vi "Export.vi"(8 "error in (no error)":errorcluster, 11 "Project Path":path) -> (0 "error out":errorcluster)   [LabVIEW 2015, in "Project.lvclass"]
uses:
  Project.lvclass
  Elemental IO Properties.ctl
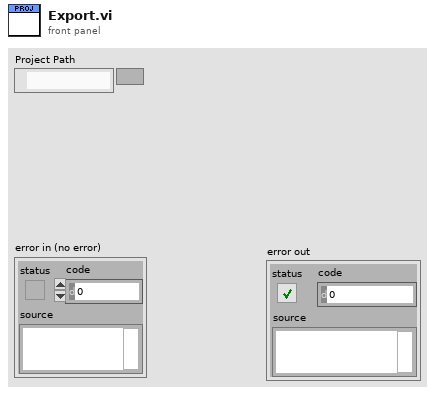
[diagram p1: front panel]
types:
  T1 = enum16{"open", "replace", "create", "open or create", "replace or create", "replace or create with confirmation"}
  T2 = typedef "Project.lvclass/Elemental IO Properties.ctl" = cluster{"FPGA":string, "Mod":string, "IO Resource":string, "IO Name":string}
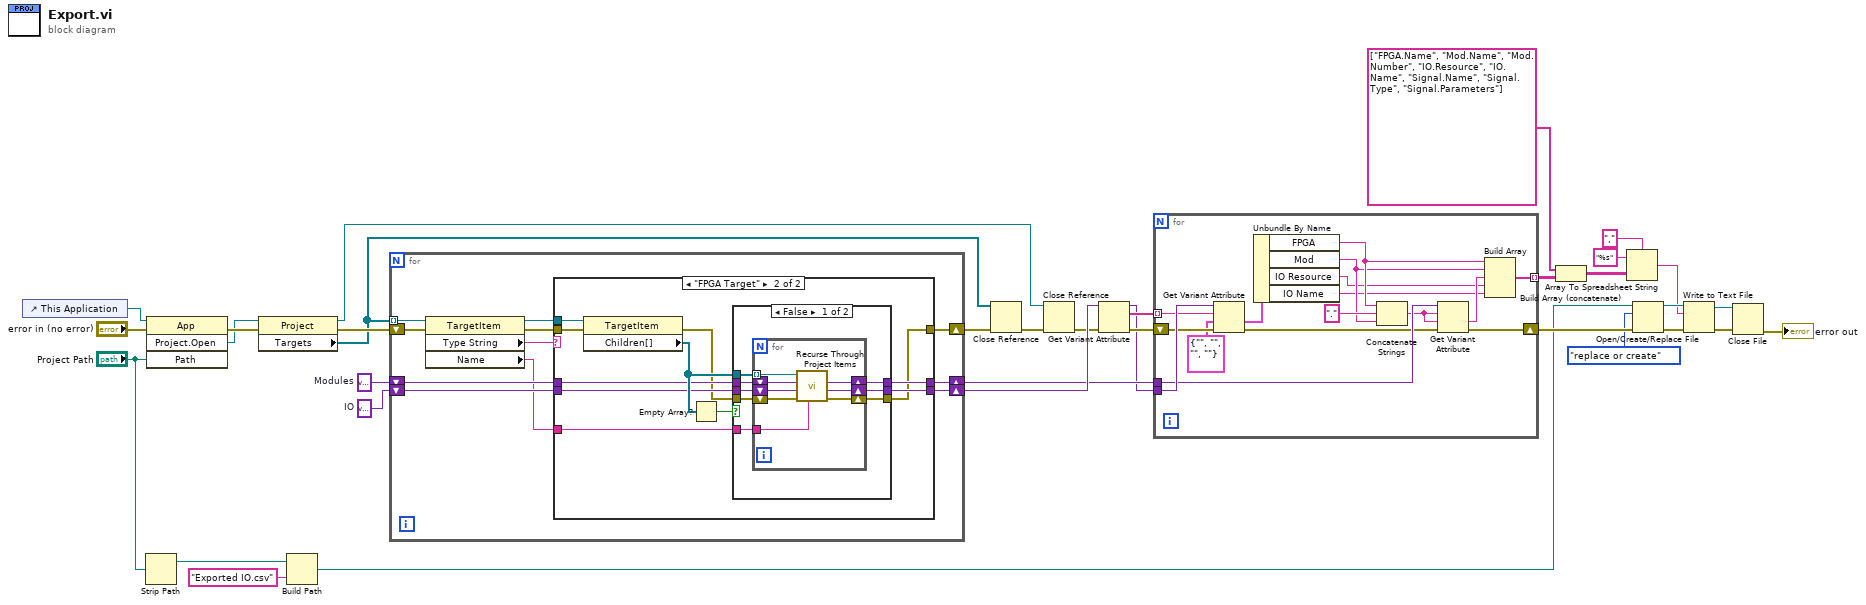
[diagram p0: block diagram]
diagram:
  w25 = variant  # IO
  w26 = variant  # Modules
  n1 = control-ref of="This Application"() -> (w34:refnum<vi>)
  n2 = Strip Path(path="Project Path") -> (stripped path=w6:path)  [unwired: 1 out]
  n3 = invoke class="App" method="Project.Open"(reference=w34, error in="error in (no error)", "Path"="Project Path") -> (error out=w33:errorcluster, "Project:Open"=w32:refnum<vi>)  [unwired: 1 in, 2 out]
  n4 = property class="Project"(reference=w32, error in=w33) -> (reference out=w28:refnum<vi>, error out=w31:errorcluster, "Targets"=w29:refnum<vi>[])
  n5 = Build Path(base path=w6, name or relative path="Exported IO.csv") -> (appended path=w3:path)
  n6 = for {
    tunnel: w29 -> [w45] mode=indexing
    shift-right: [w42] -> w30
    shift-left: w31 -> [w44]
    shift-right: [w39] -> w22
    shift-left: w26 -> [w40]
    shift-right: [w37] -> w23
    shift-left: w25 -> [w38]
    n7 = property class="TargetItem"(reference=w45, error in=w44) -> (reference out=w41:refnum<vi>, error out=w43:errorcluster, "Type String"=w36:string, "Name"=w35:string)
    n8 = case shown="\"FPGA Target\"" w36 {
      tunnel: w43 -> [w48 w59]
      tunnel: [w48 w49] -> w42
      tunnel: w41 -> [_ w58]
      tunnel: w40 -> [w47 w55]
      tunnel: w35 -> [_ w54]
      tunnel: [w47 w53] -> w39
      tunnel: w38 -> [w46 w52]
      tunnel: [w46 w51] -> w37
      frame "False", Default {
      }
      frame "FPGA Target" {
        n9 = property class="TargetItem"(reference=w58, error in=w59) -> (error out=w50:errorcluster, "Children[]"=w57:refnum<vi>[])  [unwired: 1 out]
        n10 = Empty Array?(array=w57) -> (empty?=w56:bool)
        n11 = case shown="False" w56 {
          tunnel: w57 -> [w67 _]
          tunnel: w50 -> [w66 w76]
          tunnel: w55 -> [w65 w78]
          tunnel: w54 -> [w64 _]
          tunnel: [w63 w78] -> w53
          tunnel: w52 -> [w62 w77]
          tunnel: [w61 w77] -> w51
          tunnel: [w60 w76] -> w49
          frame False {
            n12 = for {
              tunnel: w67 -> [w75] mode=indexing
              shift-right: [w73] -> w60
              shift-left: w66 -> [w74]
              shift-right: [w72] -> w63
              shift-left: w65 -> [w69]
              tunnel: w64 -> [w68]
              shift-right: [w71] -> w61
              shift-left: w62 -> [w70]
              n13 = call "Recurse Through Project Items.vi"("FPGA"=w68, "error in (no error)"=w74, "IO in"=w70, "Modules in"=w69, "ProjectItem in"=w75) -> ("error out"=w73:errorcluster, "IO out"=w71:variant, "Modules out"=w72:variant)  [unwired: 4 in]
            }
          }
          frame True {
          }
        }
      }
    }
  }
  n14 = Close Reference(reference=w29, error in (no error)=w30) -> (error out=w27:errorcluster)
  n15 = Close Reference(reference=w28, error in (no error)=w27) -> (error out=w20:errorcluster)
  n16 = Get Variant Attribute(Variant=w23, error in=w20) -> (duplicate Variant=w18:variant, names=w24:string[], error out=w21:errorcluster)  [unwired: 2 in, 1 out]
  n17 = for {
    tunnel: w24 -> [w81] mode=indexing
    tunnel: w18 -> [w94]
    tunnel: w22 -> [w93]
    tunnel: [w84] -> w1 mode=indexing
    shift-right: [w83] -> w12
    shift-left: w21 -> [w89]
    n18 = Get Variant Attribute(Variant=w94, name=w81, default value (empty Variant)=T2 {"FPGA"="", "Mod"="", "IO Resource"="", "IO Name"=""}, error in=w89) -> (value=w92:T2, error out=w90:errorcluster)  [unwired: 2 out]
    n19 = Unbundle By Name(w92) -> ("FPGA"=w88:string, "Mod"=w87:string, "IO Resource"=w85:string, "IO Name"=w80:string)
    n20 = Concatenate Strings(w88, "." ("string"), w87) -> (w82:string)
    n21 = Get Variant Attribute(Variant=w93, name=w82, default value (empty Variant)=w82, error in=w90) -> (value=w86:string, error out=w83:errorcluster)  [unwired: 2 out]
    n22 = Build Array(w88, w87, w86, w85, w80) -> (w84:string[])
  }
  n23 = Build Array (concatenate)(string[] ["FPGA.Name", "Mod.Name", "Mod.Number", "IO.Resource", "IO.Name", "Signal.Name", "Signal.Type", "Signal.Parameters"] ("names"), w1) -> (w2:string[][])
  n24 = Array To Spreadsheet String(delimiter (Tab)=",", array=w2, 3:"%s" ("format string")) -> (spreadsheet string=w8:string)
  n25 = Open/Create/Replace File(file path (use dialog)=w3, error in=w12, operation (0:open)=T1."replace or create") -> (refnum out=w13:refnum<file>, error out=w14:errorcluster)  [unwired: 3 in, 1 out]
  n26 = Write to Text File(file (use dialog)=w13, text=w8, error in=w14) -> (refnum out=w10:refnum<file>, error out=w11:errorcluster)  [unwired: 1 in, 1 out]
  n27 = Close File(refnum=w10, error in=w11) -> (error out=→"error out":errorcluster)  [unwired: 1 out]
